vi "Read Invidual Beams.vi"(8 "error in (no error)":errorcluster, 11 "Toggle 8 in":refnum<class "Toggle 8.lvclass">) -> (0 "error out":errorcluster, 2 "Invidual Beams":u8[][](array[numeric])=[[0, 0], [64, 0], [32, 0], [16, 0], [8, 0], [4, 0], [2, 0], [1, 0], [0, 64], [0, 32], [0, 16], [0, 8], [0, 4], [0, 2], [0, 1]] format="%x", 3 "Toggle 8 out":refnum<class "Toggle 8.lvclass">)   [LabVIEW 2020, in "Toggle 8.lvclass"]
uses:
  Toggle 8.lvclass
  Toggle 8.lvclass/Toggle 8.ctl
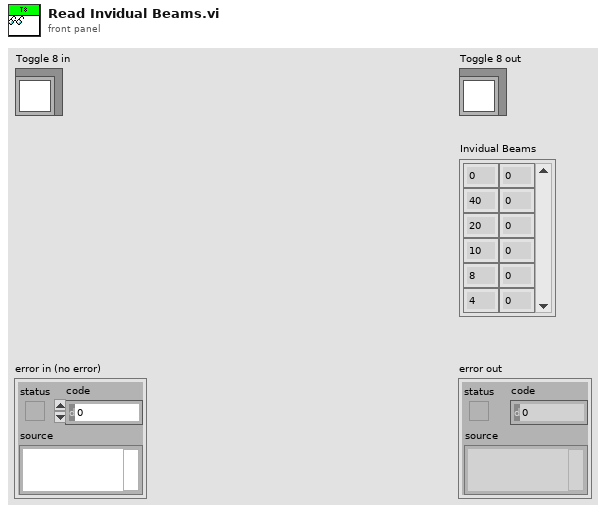
[diagram p1: front panel]
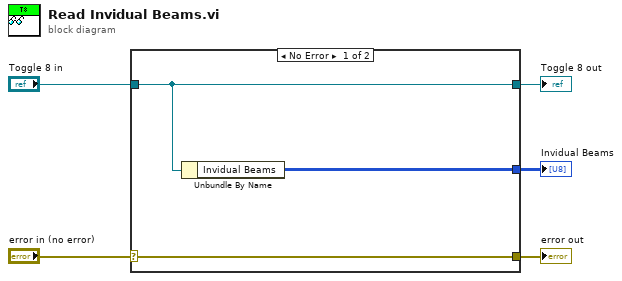
[diagram p0: block diagram]
diagram:
  n1 = case shown="No Error" "error in (no error)" {
    selector: "error in (no error)" -> [w8 w9]
    tunnel: [w8 w9] -> w4
    tunnel: [w7 w10] -> w2
    tunnel: "Toggle 8 in" -> [w7 w10]
    tunnel: [w6 _] -> w1
    frame No Error {
      n2 = Unbundle By Name(w7) -> ("Invidual Beams"=w6:u8[][])
    }
    frame Error {
    }
  }
  "error out" <- w4
  "Toggle 8 out" <- w2
  "Invidual Beams" <- w1
